vi "HelperVI1-array.vi"() -> ()   [LabVIEW 2016, in "test_ValueSignal.lvlib"]
uses:
  test_ValueSignal.lvlib
panel:
  in  "String array":string[](array[string])
  in  "Numeric array":dbl[](array[numeric])
  in  "Cluster array":T1(array[cluster])
  in  "Boolean array":bool[](array[boolean])
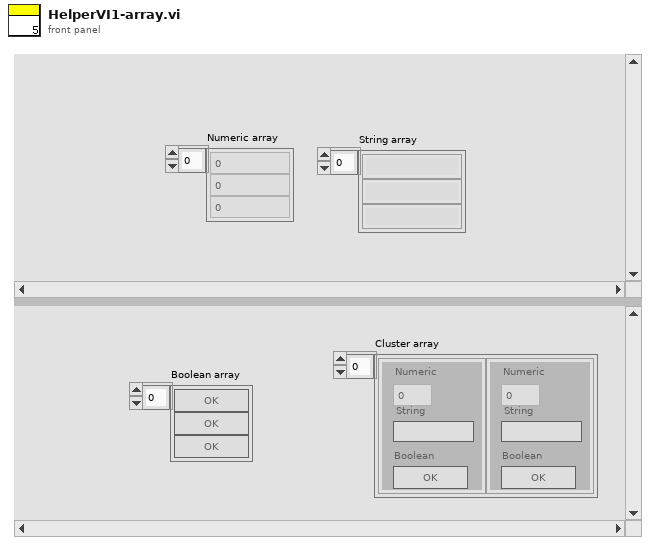
[diagram p1: front panel]
types:
  T1 = cluster{"Numeric":dbl, "String":string, "Boolean":bool}[]
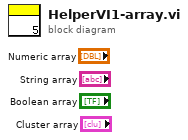
[diagram p0: block diagram]
diagram:
